vi "运行间隔计算.vi"(11 "运行周期":i16=4) -> (3 "数组":i32[](array[numeric]))   [LabVIEW 2016, in "PLC.lvlib"]
uses:
  PLC.lvlib
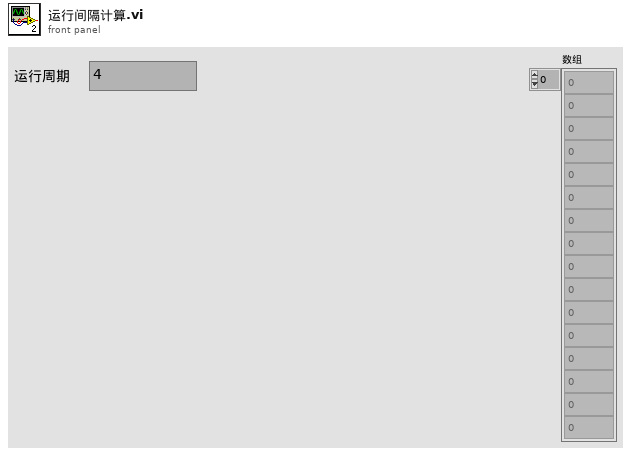
[diagram p1: front panel]
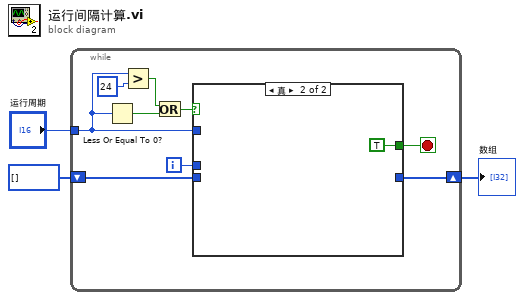
[diagram p0: block diagram]
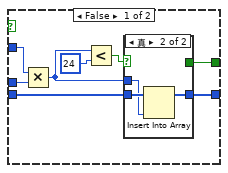
[diagram p2: hidden frame]
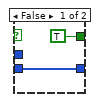
[diagram p3: hidden frame]
diagram:
  n1 = while {
    tunnel: "运行周期" -> [w7]
    shift-right: [w10] -> w1
    shift-left: i32[] [] -> [w11]
    i -> [w12]
    stop <- w9 stop-if-true
    n2 = Less Or Equal To 0?(x=w7) -> (x <= 0?=w6:bool)
    n3 = Greater?(x=w7, y=i16 24) -> (0:w5:bool)
    n4 = Or(x=w5, y=w6) -> (x .or. y?=w4:bool)
    n5 = case shown="真" w4 {
      tunnel: w12 -> [w20 _]
      tunnel: w11 -> [w19 _]
      tunnel: [w18 _] -> w10
      tunnel: [w15 TRUE] -> w9
      tunnel: w7 -> [w13 _]
      frame False {
        n6 = Multiply(x=w13, y=w20) -> (x*y=w14:i32)
        n7 = Less?(x=w14, y=24) -> (x < y?=w16:bool)
        n8 = case shown="真" w16 {
          tunnel: w19 -> [w22 w25]
          tunnel: [w22 w24] -> w18
          tunnel: [TRUE _] -> w15
          tunnel: w14 -> [_ w23]
          frame False {
          }
          frame True {
            n9 = Insert Into Array(array=w25, new element=w23) -> (w24:i32[])  [unwired: 1 in]
          }
        }
      }
      frame True {
      }
    }
  }
  "数组" <- w1
